vi "Read File.vi"(8 "error in (no error)":errorcluster, 10 "Parameters":refnum<class "Parameter.lvclass">[](array[class]), 11 "Parameter INI File in":refnum<class "Parameter INI File.lvclass">) -> (0 "error out":errorcluster, 2 "Parameters":refnum<class "Parameter.lvclass">[](array[class]), 3 "Parameter INI File out":refnum<class "Parameter INI File.lvclass">)   [LabVIEW 2016, in "CD Parameter Manager API.lvlib" / "Parameter INI File.lvclass"]
uses:
  Parameter INI File.lvclass
  <vilib>/Utility/config.llb/NI_LVConfig.lvlib
  <vilib>/Utility/error.llb/Error Cluster From Error Code.vi
  <vilib>/ErrorRing/Error Ring.xnode
  Boolean Parameter Class/Boolean Parameter.lvclass
  I32 Parameter Class/I32 Parameter.lvclass
  <vilib>/Utility/config.llb/Read Key (Boolean).vi
  <vilib>/Utility/config.llb/Read Key (I32).vi
  Double Parameter Class/Double Parameter.lvclass
  <vilib>/Utility/config.llb/Read Key (Double).vi
  String Parameter Class/String Parameter.lvclass
  <vilib>/Utility/config.llb/Read Key (String).vi
  Parameter Class/Parameter.lvclass
  C:/Repositories/UI-Control-Initializer-API/Source/Parameter Class/Parameter.lvclass
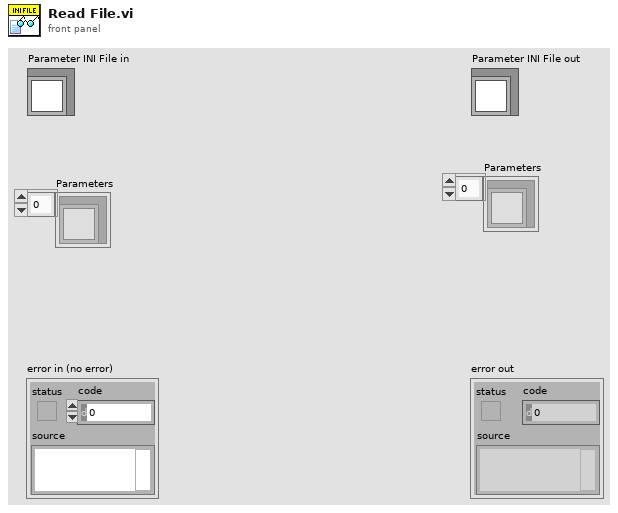
[diagram p1: front panel]
types:
  T1 = typedef "NI_LVConfig.lvlib/Config Data RefNum.ctl" = refnum<k1>
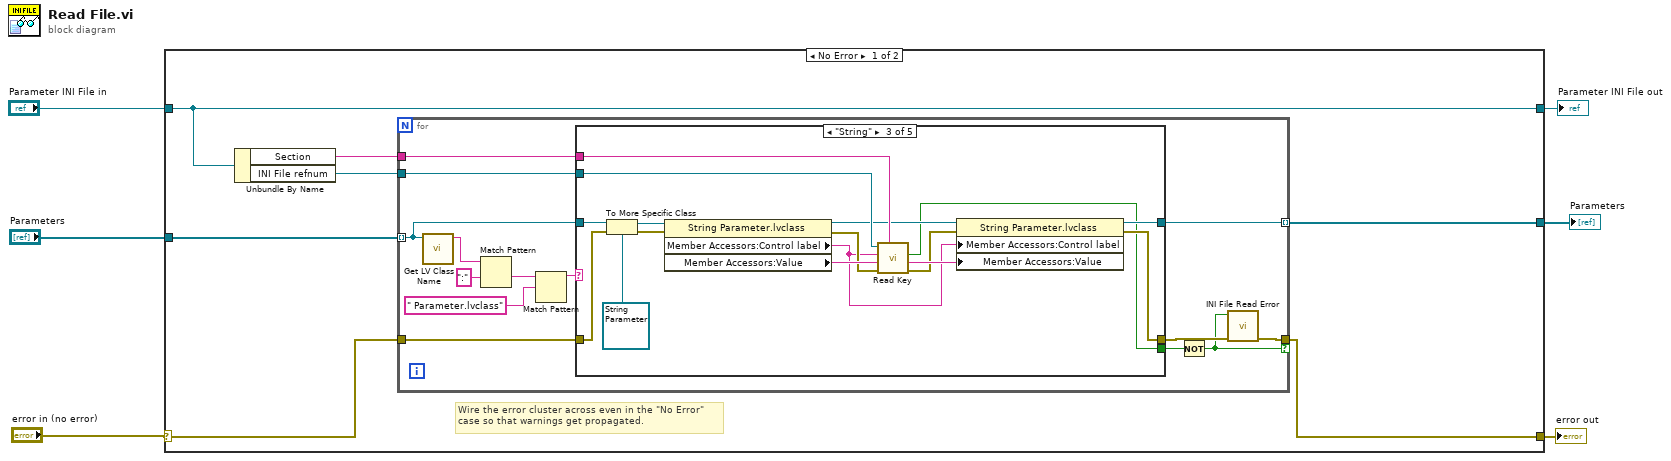
[diagram p0: block diagram]
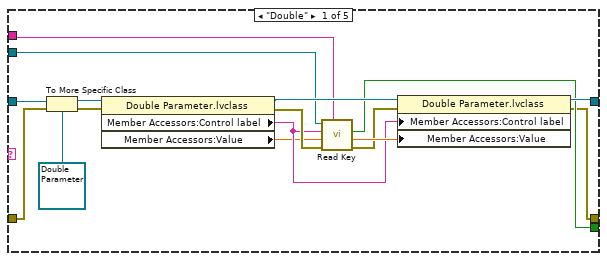
[diagram p2: hidden frame]
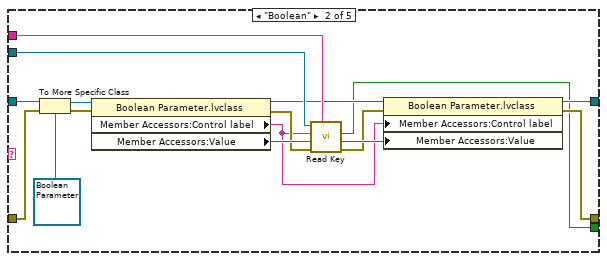
[diagram p3: hidden frame]
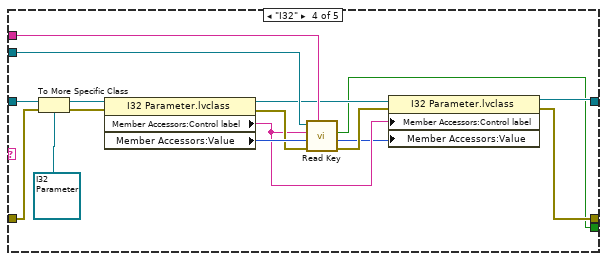
[diagram p4: hidden frame]
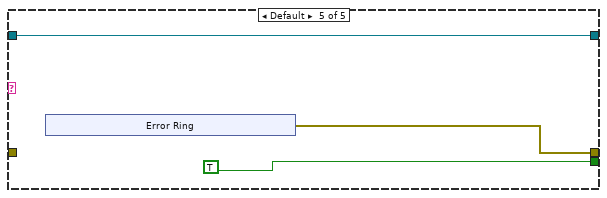
[diagram p5: hidden frame]
diagram:
  n1 = case shown="No Error" "error in (no error)" {
    selector: "error in (no error)" -> [w13 w102]
    tunnel: [w8 w102] -> w4
    tunnel: [w10 w101] -> w5
    tunnel: "Parameter INI File in" -> [w10 w101]
    tunnel: "Parameters" -> [w9 w100]
    tunnel: [w7 w100] -> w1
    frame No Error {
      # "Wire the error cluster across even in the \"No Error\"\ncase so that warnings get propagated."
      n2 = Unbundle By Name(w10) -> ("Section"=w11:string, "INI File refnum"=w12:T1)
      n3 = for {
        tunnel: w13 -> [w22]
        tunnel: [w15] -> w8 if=w14
        tunnel: w12 -> [w20]
        tunnel: w9 -> [w19] mode=indexing
        tunnel: w11 -> [w18]
        tunnel: [w17] -> w7 mode=indexing
        n4 = call <vilib>:"Get LV Class Name.vi"("object"=w19) -> ("class name"=w24:string)  [unwired: 9 in, 1 out]
        n5 = Match Pattern(string=w24, regular expression=":") -> (after substring=w26:string)  [unwired: 1 in, 3 out]
        n6 = Match Pattern(string=w26, regular expression=" Parameter.lvclass") -> (before substring=w23:string)  [unwired: 1 in, 3 out]
        n7 = case shown="\"String\"" w23 {
          tunnel: w22 -> [w39 w55 w71 w87 _]
          tunnel: [w30 w46 w63 w78 w93] -> w16
          tunnel: [w31 w44 w61 w76 TRUE] -> w21
          tunnel: w20 -> [w28 w52 w68 w85 _]
          tunnel: w19 -> [w42 w56 w72 w88 w92]
          tunnel: w18 -> [w29 w53 w69 w84 _]
          tunnel: [w32 w45 w62 w81 w92] -> w17
          frame "Double" {
            n8 = To More Specific Class(target class=refnum<class "Double Parameter.lvclass"> refnum ("CD Parameter Manager API.lvlib:Double Parameter.lvclass"), reference=w42, error in=w39) -> (specific class reference=w41:refnum<class "Double Parameter.lvclass">, error out=w43:errorcluster)
            n9 = property class="Double Parameter.lvclass"(reference=w41, error in=w43) -> (reference out=w36:refnum<class "Double Parameter.lvclass">, error out=w35:errorcluster, "Member Accessors:Control label"=w34:string, "Member Accessors:Value"=w33:dbl)
            n10 = call-poly <vilib>:"Read Key.vi"("section"=w29, "error in (no error)"=w35, "default value"=w33, "key"=w34, "refnum"=w28) -> ("error out"=w37:errorcluster, "value"=w38:dbl, "found?"=w31:bool)  [unwired: 3 in, 1 out]
            n11 = property class="Double Parameter.lvclass"(reference=w36, error in=w37, "Member Accessors:Control label"=w34, "Member Accessors:Value"=w38) -> (reference out=w32:refnum<class "Double Parameter.lvclass">, error out=w30:errorcluster)
          }
          frame "Boolean" {
            n12 = To More Specific Class(target class=refnum<class "Boolean Parameter.lvclass"> refnum ("CD Parameter Manager API.lvlib:Boolean Parameter.lvclass"), reference=w56, error in=w55) -> (specific class reference=w58:refnum<class "Boolean Parameter.lvclass">, error out=w59:errorcluster)
            n13 = property class="Boolean Parameter.lvclass"(reference=w58, error in=w59) -> (reference out=w48:refnum<class "Boolean Parameter.lvclass">, error out=w54:errorcluster, "Member Accessors:Control label"=w47:string, "Member Accessors:Value"=w57:bool)
            n14 = call-poly <vilib>:"Read Key.vi"("section"=w53, "error in (no error)"=w54, "default value"=w57, "key"=w47, "refnum"=w52) -> ("error out"=w49:errorcluster, "value"=w50:bool, "found?"=w44:bool)  [unwired: 3 in, 1 out]
            n15 = property class="Boolean Parameter.lvclass"(reference=w48, error in=w49, "Member Accessors:Control label"=w47, "Member Accessors:Value"=w50) -> (reference out=w45:refnum<class "Boolean Parameter.lvclass">, error out=w46:errorcluster)
          }
          frame "String" {
            n16 = To More Specific Class(target class=refnum<class "String Parameter.lvclass"> refnum ("CD Parameter Manager API.lvlib:String Parameter.lvclass"), reference=w72, error in=w71) -> (specific class reference=w74:refnum<class "String Parameter.lvclass">, error out=w75:errorcluster)
            n17 = property class="String Parameter.lvclass"(reference=w74, error in=w75) -> (reference out=w65:refnum<class "String Parameter.lvclass">, error out=w70:errorcluster, "Member Accessors:Control label"=w64:string, "Member Accessors:Value"=w73:string)
            n18 = call-poly <vilib>:"Read Key.vi"("section"=w69, "error in (no error)"=w70, "default value"=w73, "key"=w64, "refnum"=w68) -> ("error out"=w66:errorcluster, "value"=w67:string, "found?"=w61:bool)  [unwired: 3 in, 1 out]
            n19 = property class="String Parameter.lvclass"(reference=w65, error in=w66, "Member Accessors:Control label"=w64, "Member Accessors:Value"=w67) -> (reference out=w62:refnum<class "String Parameter.lvclass">, error out=w63:errorcluster)
          }
          frame "I32" {
            n20 = To More Specific Class(target class=refnum<class "I32 Parameter.lvclass"> refnum ("CD Parameter Manager API.lvlib:I32 Parameter.lvclass"), reference=w88, error in=w87) -> (specific class reference=w90:refnum<class "I32 Parameter.lvclass">, error out=w91:errorcluster)
            n21 = property class="I32 Parameter.lvclass"(reference=w90, error in=w91) -> (reference out=w82:refnum<class "I32 Parameter.lvclass">, error out=w86:errorcluster, "Member Accessors:Control label"=w79:string, "Member Accessors:Value"=w89:i32)
            n22 = call-poly <vilib>:"Read Key.vi"("section"=w84, "error in (no error)"=w86, "default value"=w89, "key"=w79, "refnum"=w85) -> ("error out"=w80:errorcluster, "value"=w77:i32, "found?"=w76:bool)  [unwired: 3 in, 1 out]
            n23 = property class="I32 Parameter.lvclass"(reference=w82, error in=w80, "Member Accessors:Control label"=w79, "Member Accessors:Value"=w77) -> (reference out=w81:refnum<class "I32 Parameter.lvclass">, error out=w78:errorcluster)
          }
          frame Default {
            n24 = xnode "Error Ring"() -> ("error out"=w93:errorcluster)
          }
        }
        n25 = Not(x=w21) -> (.not. x?=w14:bool)
        n26 = call "INI File Read Error.vi"("error in (no error)"=w16, "INI Key Not Found?"=w14) -> ("error out"=w15:errorcluster)  [unwired: 9 in]
      }
    }
    frame Error {
    }
  }
  "error out" <- w4
  "Parameter INI File out" <- w5
  "Parameters" <- w1
